vi "UTF8 issues tests.vi"() -> ()   [LabVIEW 2017]
panel:
  out "string":string
  out "error out":errorcluster
  out "time":dbl format="%#_3p"
  out "utf-8 text":string
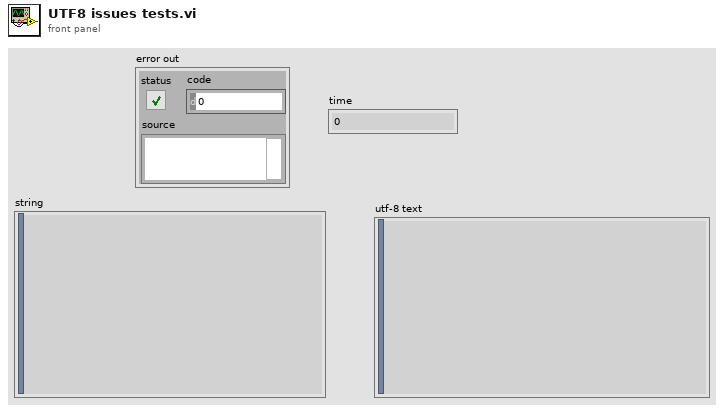
[diagram p1: front panel]
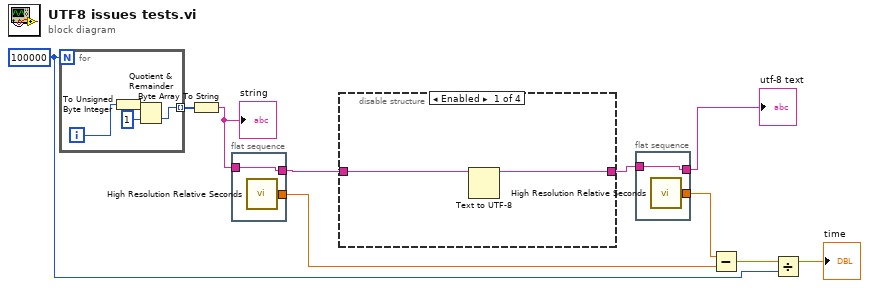
[diagram p0: block diagram]
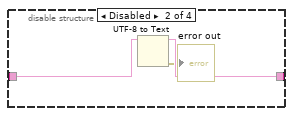
[diagram p2: hidden frame]
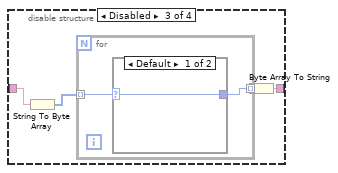
[diagram p3: hidden frame]
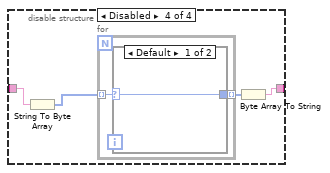
[diagram p5: hidden frame]
diagram:
  w1 = 100000
  n1 = for {
    N: w1 -> [_]
    tunnel: [w11] -> w10 mode=indexing
    i -> [w14]
    n2 = To Unsigned Byte Integer(number=w14) -> (unsigned 8bit integer=w13:u8)
    n3 = Quotient & Remainder(x=w13, y=u8 1) -> (floor(x/y)=w11:u8)  [unwired: 1 out]
  }
  n4 = Byte Array To String(unsigned byte array=w10) -> (string=w9:string)
  "string" <- w9
  n5 = flat-sequence {
    tunnel: w9 -> [w16]
    tunnel: [w16] -> w8
    tunnel: [w15] -> w4
    frame #0 {
      n6 = call <vilib>:"High Resolution Relative Seconds.vi"() -> ("relative seconds"=w15:dbl)
    }
  }
  n7 = disable-structure shown="Enabled" {
    disable-tunnel: w8 -> [w18 w21 w24 w33]
    disable-tunnel: [w17 w20 w22 w30] -> w7
    frame Enabled {
      n8 = Text to UTF-8(11:w18) -> (3:w17:string)  [unwired: 2 in, 1 out]
    }
    frame Disabled {
      n9 = UTF-8 to Text(11:w21) -> (0:→"error out":errorcluster, 3:w20:string)  [unwired: 2 in]
    }
    frame Disabled {
      n10 = String To Byte Array(string=w24) -> (unsigned byte array=w25:u8[])
      n11 = for {
        tunnel: w25 -> [w27] mode=indexing
        tunnel: [w26] -> w23 mode=indexing
        n12 = case shown="Default" w27 {
          selector: w27 -> [w28 w29]
          tunnel: [w28 w29] -> w26
          frame Default {
          }
          frame 0..127 {
          }
        }
      }
      n13 = Byte Array To String(unsigned byte array=w23) -> (string=w22:string)
    }
    frame Disabled {
      n14 = String To Byte Array(string=w33) -> (unsigned byte array=w32:u8[])
      n15 = for {
        tunnel: w32 -> [w35] mode=indexing
        tunnel: [w34] -> w31 mode=indexing
        n16 = case shown="Default" w35 {
          selector: w35 -> [w36 w37]
          tunnel: [w36 w37] -> w34
          frame Default {
          }
          frame 0..127 {
          }
        }
      }
      n17 = Byte Array To String(unsigned byte array=w31) -> (string=w30:string)
    }
  }
  n18 = flat-sequence {
    tunnel: w7 -> [w39]
    tunnel: [w39] -> w6
    tunnel: [w38] -> w5
    frame #0 {
      n19 = call <vilib>:"High Resolution Relative Seconds.vi"() -> ("relative seconds"=w38:dbl)
    }
  }
  n20 = Subtract(x=w5, y=w4) -> (x-y=w3:dbl)
  n21 = Divide(x=w3, y=w1) -> (x/y=→"time":dbl)
  "utf-8 text" <- w6
